vi "KE2657A_Test.vi"(8 "error in (no error)":errorcluster, 11 "KE2657A in":refnum<class "KE2657A.lvclass">) -> (0 "error out":errorcluster, 3 "KE2410 out":refnum<class "KE2657A.lvclass">)   [LabVIEW 2019, in "KE2657A.lvclass"]
uses:
  KE2657A.lvclass
  <vilib>/Platform/TimedLoop/XDataNode/timing_clust.ctl
  <vilib>/Platform/TimedLoop/XDataNode/nitl_modes.ctl
  <vilib>/Platform/TimedLoop/XDataNode/wakeup.ctl
  InstrumentSetup.vi
  <vilib>/platform/TimedLoop/XDataNode/XDataNode.xnode
  <vilib>/Platform/TimedLoop/XDataNode/XDNodeRunTimeDep.lvlib
  InstrControl.lvclass
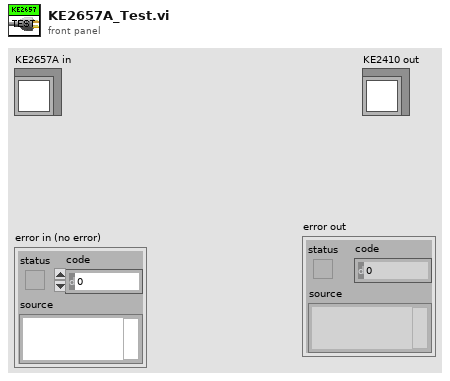
[diagram p1: front panel]
types:
  T1 = cluster{"Current Limit":sgl, "KE2657A":refnum<class "KE2657A.lvclass">}
  T2 = cluster{"KE 2410":cluster{"Instrument name":string, "address":refnum<visa-resource-name>, "Instrument type":u16}, "KE 6517":cluster{"Instrument name":string, "address":refnum<visa-resource-name>, "Instrument type":u16}, "KE 487":cluster{"Instrument name":string, "address":refnum<visa-resource-name>, "Instrument type":u16}, "KE 236":cluster{"Instrument name":string, "address":refnum<visa-resource-name>, "Instrument type":u16}, "WK 6440B":cluster{"Instrument name":string, "address":refnum<visa-resource-name>, "Instrument type":u16}, "WK 6425":cluster{"Instrument name":string, "address":refnum<visa-resource-name>, "Instrument type":u16}, "Pickering Matrix":cluster{"Instrument name":string, "address":refnum<visa-resource-name>, "Instrument type":u16}, "KE 2000":cluster{"Instrument name":string, "address":refnum<visa-resource-name>, "Instrument type":u16}, "KE3706A Switching":cluster{"Instrument name":string, "address":refnum<visa-resource-name>, "Instrument type":u16}, "KE 2657A":cluster{"Instrument name":string, "address":refnum<visa-resource-name>, "Instrument type":u16}}
  T3 = typedef "XDNodeRunTimeDep.lvlib/timing_clust.ctl" = cluster{"Expected End [f-1]":u64, "Actual End [f-1]":u64, "Finished Late? [f-1]":bool, "Expected End [i-1]":u64, "Actual End [i-1]":u64, "Finished Late? [i-1]":bool, "Expected Start [i]":u64, "Actual Start [i]":u64, "Expected Start [f]":u64, "Actual Start [f]":u64, "Source Name":string, "Structure Name":string, "Period":i64, "Deadline":i64, "Offset":i64, "Start":i64, "Priority":i32, "Timeout":i32, "Mode":T4, "Wakeup Reason":T5, "Error":errorcluster, "Source Type":string, "Secondary Source Type":string, "Global End Time":u64, "Global Start Time":u64, "Frame Duration":u64, "Iteration Duration":u64, "Assigned CPU":i32, "I/O Scan Engine Mode":u32}
  T4 = typedef "XDNodeRunTimeDep.lvlib/nitl_modes.ctl" = enum32{"No Change", "Process missed periods, maintain original phase", "Discard missed periods, maintain original phase", "Process missed periods, ignore original phase", "Discard missed periods, ignore original phase"}
  T5 = typedef "XDNodeRunTimeDep.lvlib/wakeup.ctl" = enum32{"Normal", "Aborted", "Asynchronous wakeup", "Timing source error", "Timed loop error", "Timeout"}
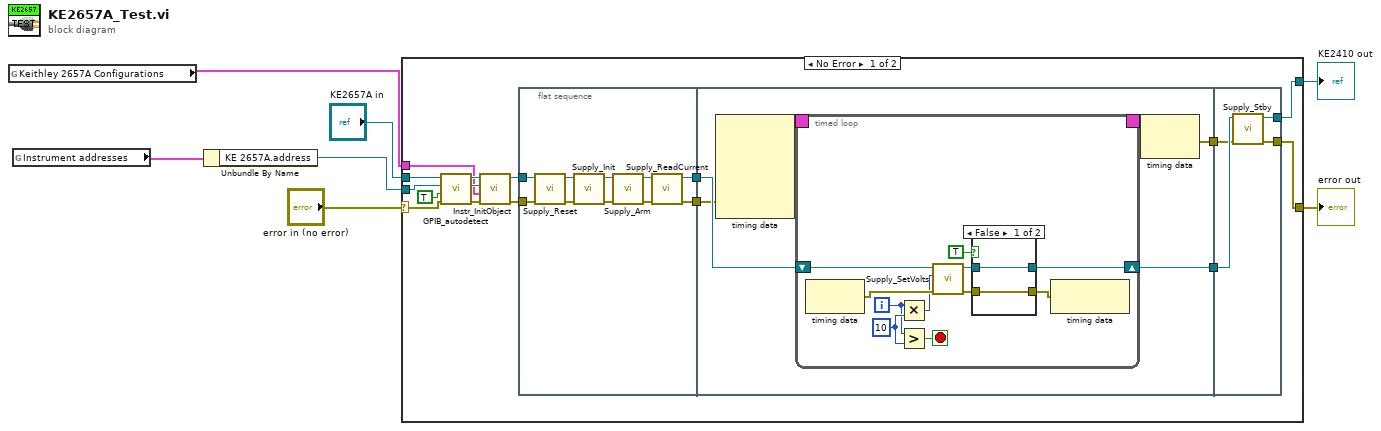
[diagram p0: block diagram]
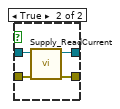
[diagram p2: hidden frame]
diagram:
  n1 = global read "InstrumentSetup.vi" "Keithley 2657A Configurations"() -> (w1:T1)
  n2 = global read "InstrumentSetup.vi" "Instrument addresses"() -> (w2:T2)
  n3 = Unbundle By Name(w2) -> ("KE 2657A.address"=w3:refnum<visa-resource-name>)
  n4 = case shown="No Error" "error in (no error)" {
    selector: "error in (no error)" -> [w18 w72]
    tunnel: "KE2657A in" -> [w16 w71]
    tunnel: [w9 w71] -> w6
    tunnel: [w20 w72] -> w5
    tunnel: w3 -> [w17 _]
    tunnel: w1 -> [w8 _]
    frame No Error {
      n5 = call-dynamic "GPIB_autodetect.vi"("error in (no error)"=w18, "Verify GPIB address"=TRUE, "Instrument address in"=w17, "InstrControl in"=w16) -> ("error out"=w13:errorcluster, "Instrument address out"=w12:refnum<visa-resource-name>, "InstrControl out"=w14:refnum<class "KE2657A.lvclass">)  [unwired: 5 in]
      n6 = call-dynamic "Instr_InitObject.vi"("error in (no error)"=w13, "Instrument Configuration"=w8, "Instrument address"=w12, "KE2657A in"=w14) -> ("error out"=w10:errorcluster, "KE2657A out"=w11:refnum<class "KE2657A.lvclass">)  [unwired: 6 in]
      n7 = flat-sequence {
        tunnel: w10 -> [w28]
        tunnel: w11 -> [w27]
        tunnel: [w25] -> w23
        tunnel: [w24] -> w19
        tunnel: w23 -> [w39]
        tunnel: [w38] -> w22
        tunnel: [w35] -> w21
        tunnel: w19 -> [w34]
        tunnel: [w68] -> w20
        tunnel: w22 -> [w69]
        tunnel: w21 -> [w70]
        tunnel: [w67] -> w9
        frame #0 {
          n8 = call-dynamic "Supply_Reset.vi"("error in (no error)"=w28, "SupplyControl in"=w27) -> ("error out"=w32:errorcluster, "SupplyControl out"=w26:refnum<class "KE2657A.lvclass">)  [unwired: 8 in]
          n9 = call-dynamic "Supply_Init.vi"("error in (no error)"=w32, "SupplyControl in"=w26) -> ("error out"=w31:errorcluster, "SupplyControl out"=w33:refnum<class "KE2657A.lvclass">)  [unwired: 8 in]
          n10 = call-dynamic "Supply_Arm.vi"("error in (no error)"=w31, "SupplyControl in"=w33) -> ("error out"=w29:errorcluster, "SupplyControl out"=w30:refnum<class "KE2657A.lvclass">)  [unwired: 8 in]
          n11 = call-dynamic "Supply_ReadCurrent.vi"("error in (no error)"=w29, "SupplyControl in"=w30) -> ("error out"=w24:errorcluster, "SupplyControl out"=w25:refnum<class "KE2657A.lvclass">)  [unwired: 7 in, 1 out]
        }
        frame #1 {
          n12 = node-c288(w34) -> (w37:T3)  [unwired: 4 in]
          n13 = timed-loop {
            timing: w37 -> [_]
            timing-out: [_] -> w36
            shift-right: [w42] -> w35
            shift-left: w39 -> [w48]
            i -> [w46]
            stop <- w45 stop-if-true
            w47 = 10
            n14 = node-c288() -> (w50:errorcluster)  [unwired: 1 in]
            n15 = Multiply(x=w46, y=w47) -> (x*y=w49:i32)
            n16 = Greater?(x=w46, y=w47) -> (0:w45:bool)
            n17 = call-dynamic "Supply_SetVolts.vi"("error in (no error)"=w50, "Volts IN [V]"=w49, "KE2657A in"=w48) -> ("error out"=w44:errorcluster, "KE2657A out"=w43:refnum<class "KE2657A.lvclass">)  [unwired: 6 in, 1 out]
            n18 = case shown="False" TRUE {
              tunnel: w44 -> [w52 w56]
              tunnel: w43 -> [w51 w55]
              tunnel: [w51 w54] -> w42
              tunnel: [w52 w53] -> w41
              frame False {
              }
              frame True {
                n19 = call-dynamic "Supply_ReadCurrent.vi"("error in (no error)"=w56, "SupplyControl in"=w55) -> ("error out"=w53:errorcluster, "SupplyControl out"=w54:refnum<class "KE2657A.lvclass">)  [unwired: 7 in, 1 out]
              }
            }
            n20 = node-c288(w41) -> ()  [unwired: 1 out]
          }
          n21 = node-c288(w36) -> (w38:errorcluster)
        }
        frame #2 {
          n22 = call-dynamic "Supply_Stby.vi"("error in (no error)"=w69, "SupplyControl in"=w70) -> ("error out"=w68:errorcluster, "SupplyControl out"=w67:refnum<class "KE2657A.lvclass">)  [unwired: 8 in]
        }
      }
    }
    frame Error {
    }
  }
  "error out" <- w5
  "KE2410 out" <- w6
